vi "Close Connection.vi"(8 "error in (no error)":errorcluster, 11 "Serial device in":refnum<class "Serial device.lvclass">) -> (0 "error out":errorcluster, 3 "Serial device out":refnum<class "Serial device.lvclass">)   [LabVIEW 2020, in "Serial device.lvclass"]
uses:
  Serial device.lvclass
  Serial device.lvclass/Serial device.ctl
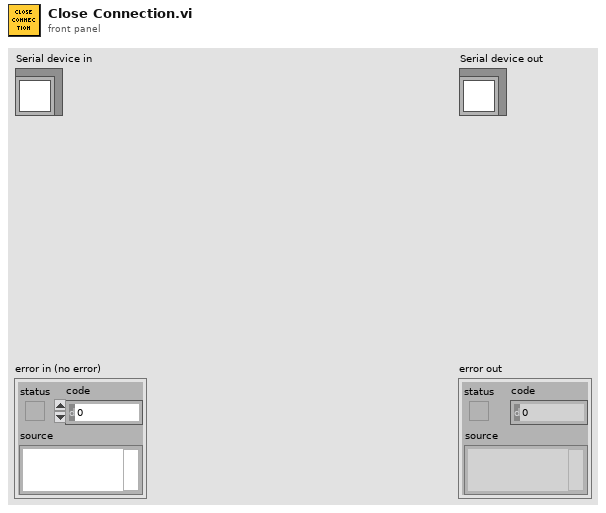
[diagram p1: front panel]
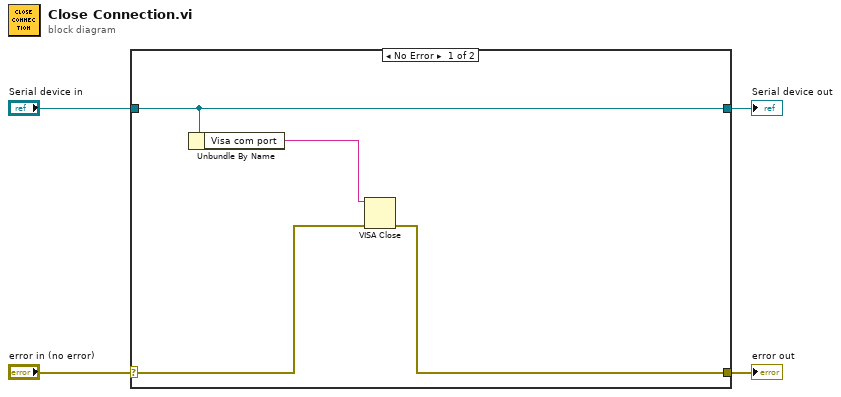
[diagram p0: block diagram]
diagram:
  n1 = case shown="No Error" "error in (no error)" {
    selector: "error in (no error)" -> [w6 w10]
    tunnel: [w5 w10] -> w3
    tunnel: [w8 w9] -> w1
    tunnel: "Serial device in" -> [w8 w9]
    frame No Error {
      n2 = Unbundle By Name(w8) -> ("Visa com port"=w7:string)
      n3 = VISA Close(VISA resource name=w7, error in (no error)=w6) -> (error out=w5:errorcluster)
    }
    frame Error {
    }
  }
  "error out" <- w3
  "Serial device out" <- w1
